vi "Configure Module.vi"(8 "error in (no error)":errorcluster, 10 "IOV ref in":variant, 11 "Module Template in":refnum<class "9217.lvclass">) -> (0 "error out":errorcluster, 2 "IOV ref out":variant, 3 "Module Template out":refnum<class "9217.lvclass">)   [LabVIEW 2019, in "Modules.lvlib" / "9217.lvclass"]
uses:
  9217.lvclass
  9217.lvclass/9217.ctl
  <resource>/objmgr/cRIO.rc
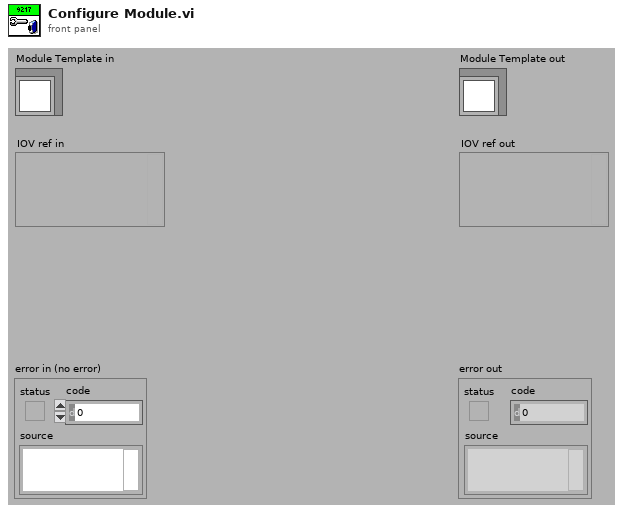
[diagram p1: front panel]
types:
  T1 = cluster{"Ohm degree range":u32, "RTD type":u32, "RTD user-defined A constant":dbl, "RTD user-defined B constant":dbl, "RTD user-defined C constant":dbl, "RTD user-defined Ro constant":dbl}[]
  T2 = cluster{"Ohm degree range":u32, "RTD type":u32, "RTD user-defined A constant":dbl, "RTD user-defined B constant":dbl, "RTD user-defined C constant":dbl, "RTD user-defined Ro constant":dbl}
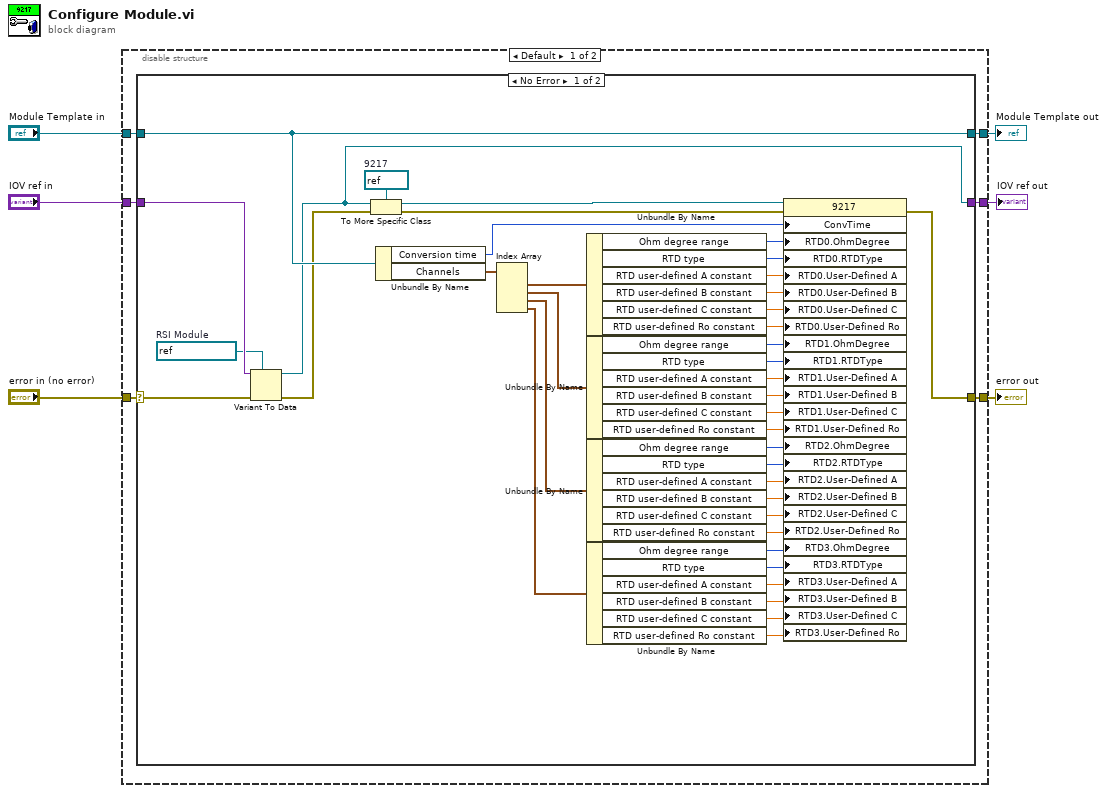
[diagram p0: block diagram]
diagram:
  n1 = disable-structure shown="Default" {
    disable-tunnel: "error in (no error)" -> [w12 w58]
    disable-tunnel: [w11 w58] -> w5
    disable-tunnel: "Module Template in" -> [w10 w56]
    disable-tunnel: [w9 w56] -> w3
    disable-tunnel: "IOV ref in" -> [w8 w57]
    disable-tunnel: [w7 w57] -> w1
    frame condition #0 (active) {
      n2 = case shown="No Error" w12 {
        selector: w12 -> [w51 w55]
        tunnel: [w47 w55] -> w11
        tunnel: [w52 w54] -> w9
        tunnel: w10 -> [w52 w54]
        tunnel: w8 -> [w15 w53]
        tunnel: [w14 w53] -> w7
        frame No Error {
          w13 = refnum<k21> refnum  # RSI Module
          w50 = refnum<k21> refnum  # 9217
          n3 = Variant To Data(error in=w51, type=w13, Variant=w15) -> (data=w14:refnum<k21>, error out=w16:errorcluster)
          n4 = To More Specific Class(target class=w50, reference=w14, error in=w16) -> (specific class reference=w49:refnum<k21>, error out=w48:errorcluster)
          n5 = Unbundle By Name(w52) -> ("Conversion time"=w46:u32, "Channels"=w45:T1)
          n6 = Index Array(array=w45) -> (element #1=w44:T2, element #2=w17:T2, element #3=w18:T2, element #4=w19:T2)  [unwired: 4 in]
          n7 = Unbundle By Name(w44) -> ("Ohm degree range"=w43:u32, "RTD type"=w42:u32, "RTD user-defined A constant"=w41:dbl, "RTD user-defined B constant"=w40:dbl, "RTD user-defined C constant"=w39:dbl, "RTD user-defined Ro constant"=w38:dbl)
          n8 = Unbundle By Name(w17) -> ("Ohm degree range"=w37:u32, "RTD type"=w36:u32, "RTD user-defined A constant"=w35:dbl, "RTD user-defined B constant"=w34:dbl, "RTD user-defined C constant"=w33:dbl, "RTD user-defined Ro constant"=w32:dbl)
          n9 = Unbundle By Name(w18) -> ("Ohm degree range"=w31:u32, "RTD type"=w30:u32, "RTD user-defined A constant"=w29:dbl, "RTD user-defined B constant"=w28:dbl, "RTD user-defined C constant"=w27:dbl, "RTD user-defined Ro constant"=w26:dbl)
          n10 = Unbundle By Name(w19) -> ("Ohm degree range"=w25:u32, "RTD type"=w24:u32, "RTD user-defined A constant"=w23:dbl, "RTD user-defined B constant"=w22:dbl, "RTD user-defined C constant"=w21:dbl, "RTD user-defined Ro constant"=w20:dbl)
          n11 = property class="9217"(reference=w49, error in=w48, "ConvTime"=w46, "RTD0.OhmDegree"=w43, "RTD0.RTDType"=w42, "RTD0.User-Defined A"=w41, "RTD0.User-Defined B"=w40, "RTD0.User-Defined C"=w39, "RTD0.User-Defined Ro"=w38, "RTD1.OhmDegree"=w37, "RTD1.RTDType"=w36, "RTD1.User-Defined A"=w35, "RTD1.User-Defined B"=w34, "RTD1.User-Defined C"=w33, "RTD1.User-Defined Ro"=w32, "RTD2.OhmDegree"=w31, "RTD2.RTDType"=w30, "RTD2.User-Defined A"=w29, "RTD2.User-Defined B"=w28, "RTD2.User-Defined C"=w27, "RTD2.User-Defined Ro"=w26, "RTD3.OhmDegree"=w25, "RTD3.RTDType"=w24, "RTD3.User-Defined A"=w23, "RTD3.User-Defined B"=w22, "RTD3.User-Defined C"=w21, "RTD3.User-Defined Ro"=w20) -> (error out=w47:errorcluster)  [unwired: 1 out]
        }
        frame Error {
        }
      }
    }
    frame condition #1 {
    }
  }
  "error out" <- w5
  "Module Template out" <- w3
  "IOV ref out" <- w1
